vi "Source DC Current.vi"(8 "error in (no error)":errorcluster, 10 "Params":variant, 11 "NI SMU in":refnum<class "NI SMU.lvclass">) -> (0 "error out":errorcluster, 3 "NI SMU out":refnum<class "NI SMU.lvclass">)   [LabVIEW 2020, in "NI SMU.lvlib" / "NI SMU.lvclass"]
uses:
  NI SMU.lvclass
  NI SMU.lvclass/NI SMU.ctl
  TypeDefs/DC current settings.ctl
  <instrlib>/niDCPower/nidcpower.llb/niDCPower Output Function.ctl
  <instrlib>/niDCPower/nidcpower.llb/niDCPower Source Mode.ctl
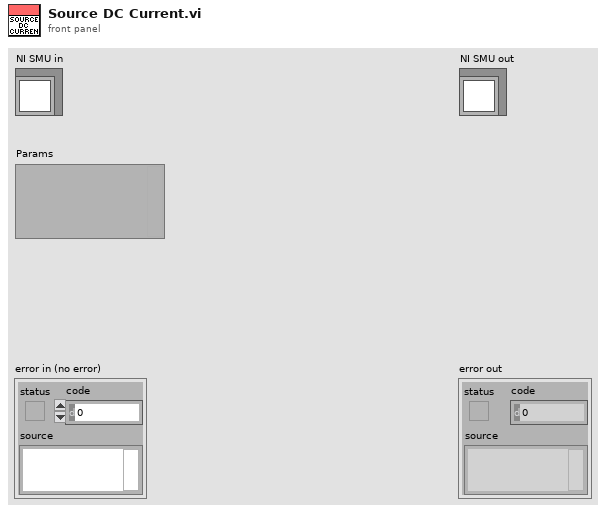
[diagram p1: front panel]
types:
  T1 = typedef "NI SMU.lvlib/NI SMU.lvclass/DC current settings.ctl" = cluster{"current level":dbl, "voltage limit":dbl, "current level range":dbl, "voltage limit range":dbl, "source delay":dbl}
  T2 = typedef "niDCPower Output Function.ctl" = i32
  T3 = typedef "niDCPower Source Mode.ctl" = i32
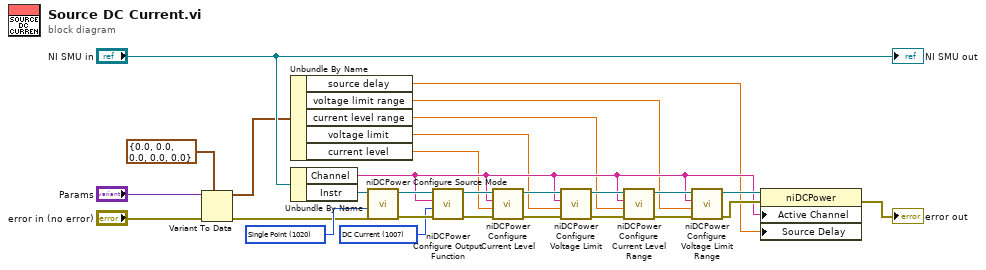
[diagram p0: block diagram]
diagram:
  w25 = T2 1007 items=["DC Voltage"=1006, "DC Current"=1007, "Pulse Voltage"=1049, "Pulse Current"=1050] ("output function")
  w26 = T3 1020 items=["Single Point"=1020, "Sequence"=1021] ("source mode")
  n1 = Variant To Data(error in="error in (no error)", type=T1 {"current level"=0.0, "voltage limit"=0.0, "current level range"=0.0, "voltage limit range"=0.0, "source delay"=0.0} ("DC current settings"), Variant="Params") -> (data=w6:T1, error out=w23:errorcluster)
  n2 = Unbundle By Name(w6) -> ("source delay"=w1:dbl, "voltage limit range"=w2:dbl, "current level range"=w3:dbl, "voltage limit"=w4:dbl, "current level"=w5:dbl)
  n3 = Unbundle By Name("NI SMU in") -> ("Channel"=w8:string, "Instr"=w24:refnum<k15>)
  n4 = call <instrlib>:"niDCPower Configure Source Mode.vi"("error in (no error)"=w23, "source mode"=w26, "instrument handle"=w24) -> ("error out"=w28:errorcluster, "instrument handle out"=w27:refnum<k15>)  [unwired: 7 out]
  n5 = call <instrlib>:"niDCPower Configure Output Function.vi"("error in (no error)"=w28, "output function"=w25, "channel name"=w8, "instrument handle"=w27) -> ("error out"=w9:errorcluster, "instrument handle out"=w15:refnum<k15>)  [unwired: 6 out]
  n6 = call <instrlib>:"niDCPower Configure Current Level.vi"("error in (no error)"=w9, "current level"=w5, "channel name"=w8, "instrument handle"=w15) -> ("error out"=w10:errorcluster, "instrument handle out"=w18:refnum<k15>)  [unwired: 6 out]
  n7 = call <instrlib>:"niDCPower Configure Voltage Limit.vi"("error in (no error)"=w10, "voltage limit"=w4, "channel name"=w8, "instrument handle"=w18) -> ("error out"=w11:errorcluster, "instrument handle out"=w17:refnum<k15>)  [unwired: 6 out]
  n8 = call <instrlib>:"niDCPower Configure Current Level Range.vi"("error in (no error)"=w11, "current level range"=w3, "channel name"=w8, "instrument handle"=w17) -> ("error out"=w12:errorcluster, "instrument handle out"=w16:refnum<k15>)  [unwired: 6 out]
  n9 = call <instrlib>:"niDCPower Configure Voltage Limit Range.vi"("error in (no error)"=w12, "voltage limit range"=w2, "channel name"=w8, "instrument handle"=w16) -> ("error out"=w13:errorcluster, "instrument handle out"=w14:refnum<k15>)  [unwired: 6 out]
  n10 = property class="niDCPower"(reference=w14, error in=w13, "Active Channel"=w8, "Source Delay"=w1) -> (error out=→"error out":errorcluster)  [unwired: 1 out]
  "NI SMU out" <- "NI SMU in"
